vi "High_Voltage_Power_Supply_Control.vi"() -> ()   [LabVIEW 2016]
uses:
  High_Voltage_Power_Supply_Control_States.ctl
  <vilib>/Utility/file.llb/Write Delimited Spreadsheet (string).vi
panel:
  in  "File Path Control":path
  in  "STOP (T = stop)":bool
  in  "COM Port In":refnum<visa-resource-name>
  in  "Measuring speed (s)":dbl=1.0 caption="Time Target (s)"
  out "Emergency Stop (T = active)":bool
  out "Connection (T = active)":bool
  in  "Control Mode (T = CV, F = CC)":bool=TRUE
  out "CH2 CURRENT OUT (mA)":dbl format="%#_4f"
  out "CH2 VOLTAGE OUT (V)":i32
  out "CH1 CURRENT OUT (mA)":dbl format="%#_4f"
  out "CH1 VOLTAGE OUT (V)":i32
  in  "CH2 CURRENT SET (0...5 mA)":dbl=5.0 min=0.0 max=5.0 step=0.1 format="%_4f"
  in  "CH1 CURRENT SET (0...5 mA)":dbl=5.0 min=0.0 max=5.0 step=0.1 format="%_4f"
  in  "CH2 VOLTAGE SET (0...+2000 V)":i16 min=0 max=2000 step=100
  in  "CH1 VOLTAGE SET (-2000...0 V)":i16 min=-2000 max=0 step=100
  in  "CH2 ON/OFF (T = ON)":bool
  in  "CH1 ON/OFF (T = ON)":bool
  # "High Voltage Power Supply"
  # "CH1: -2000...0 V"
  # "CH2: 0...+2000 V"
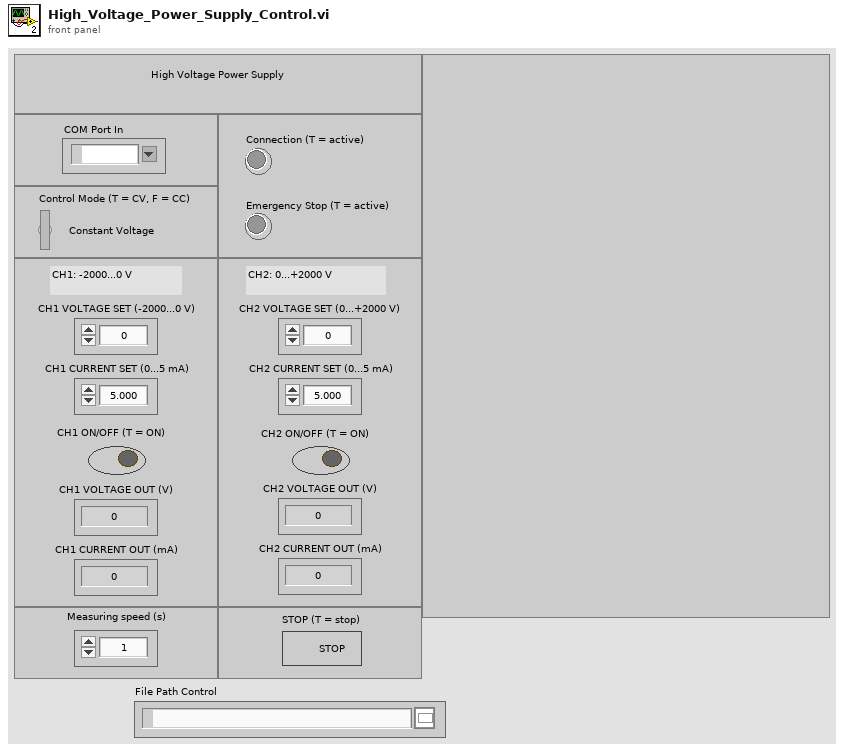
[diagram p1: front panel]
types:
  T1 = typedef "High_Voltage_Power_Supply_Control_States.ctl" = enum16{"CONTROL", "STOP", "INITIALISATION"}
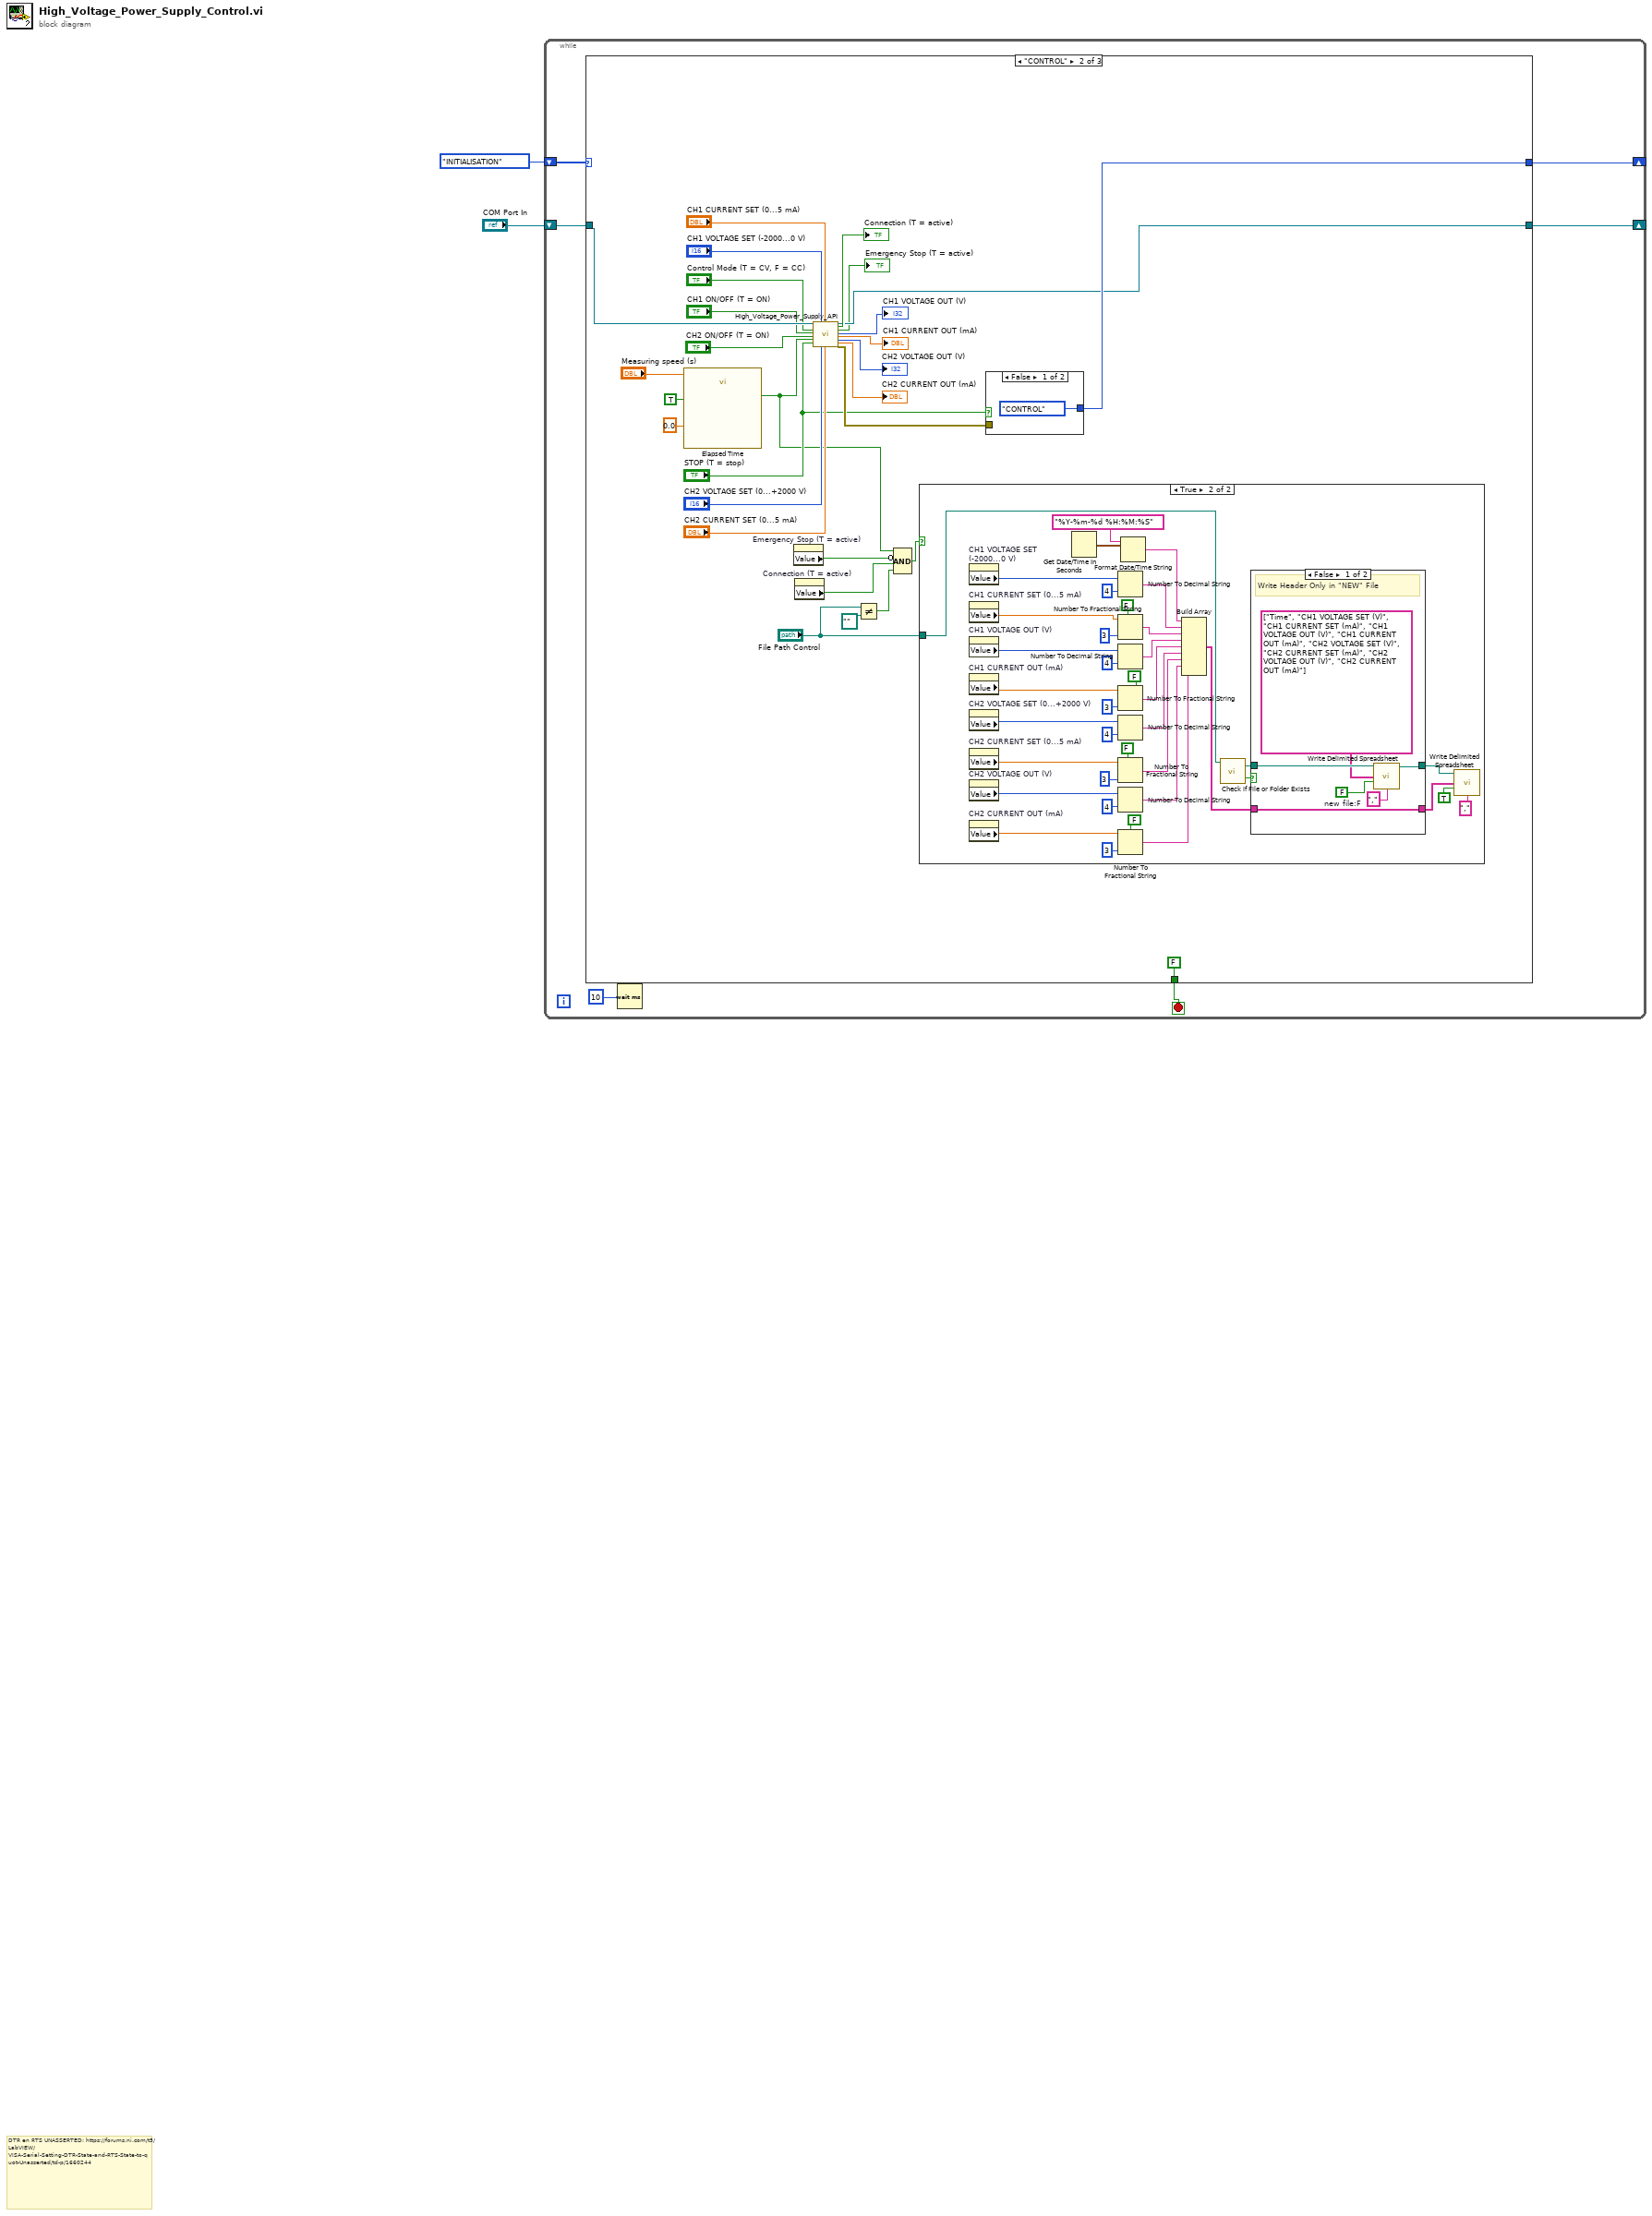
[diagram p0: block diagram]
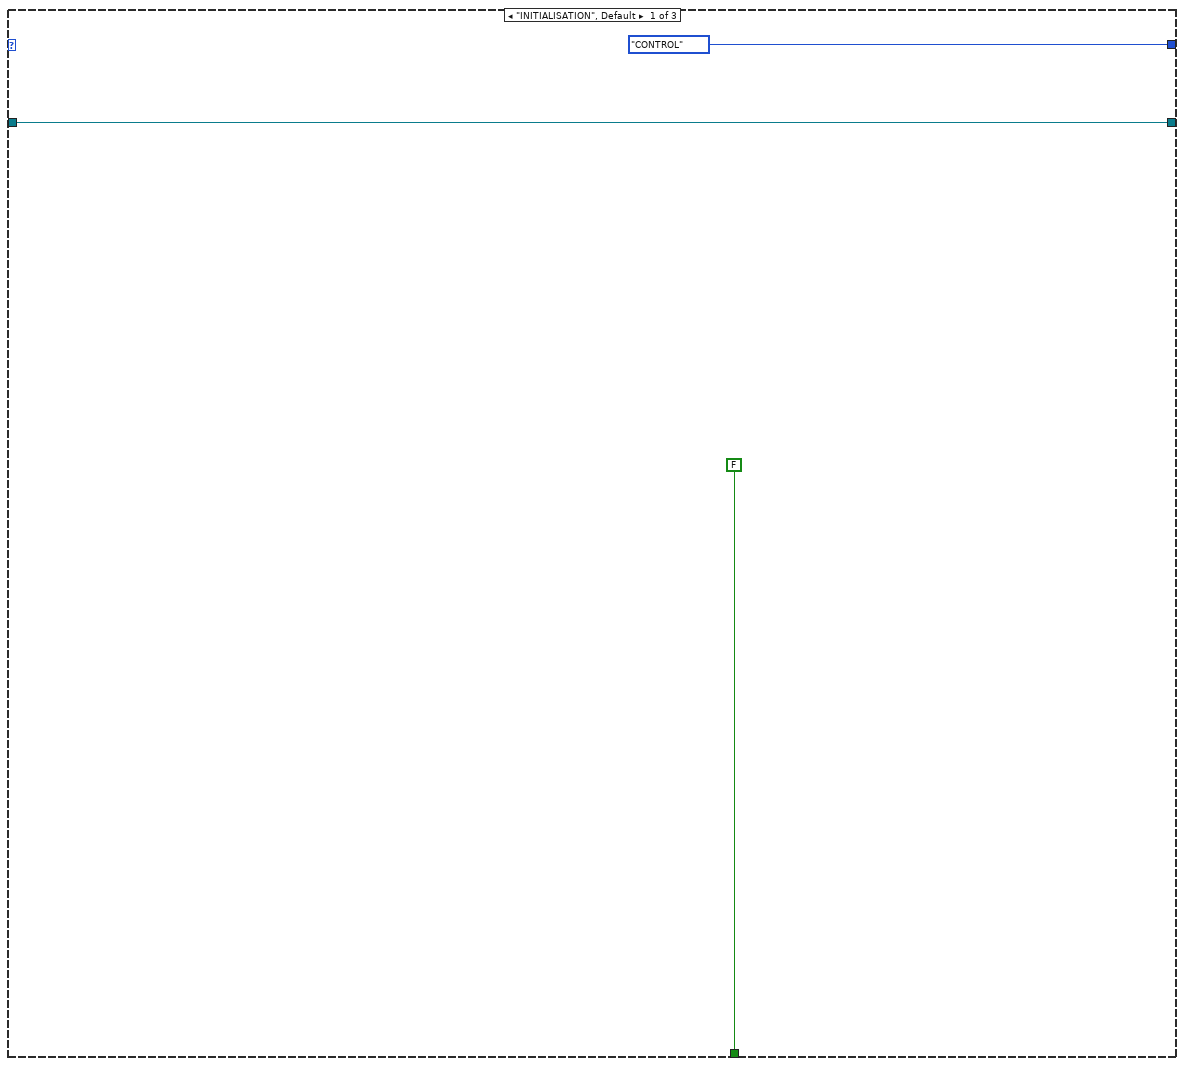
[diagram p2: hidden frame]
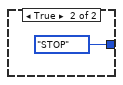
[diagram p5: hidden frame]
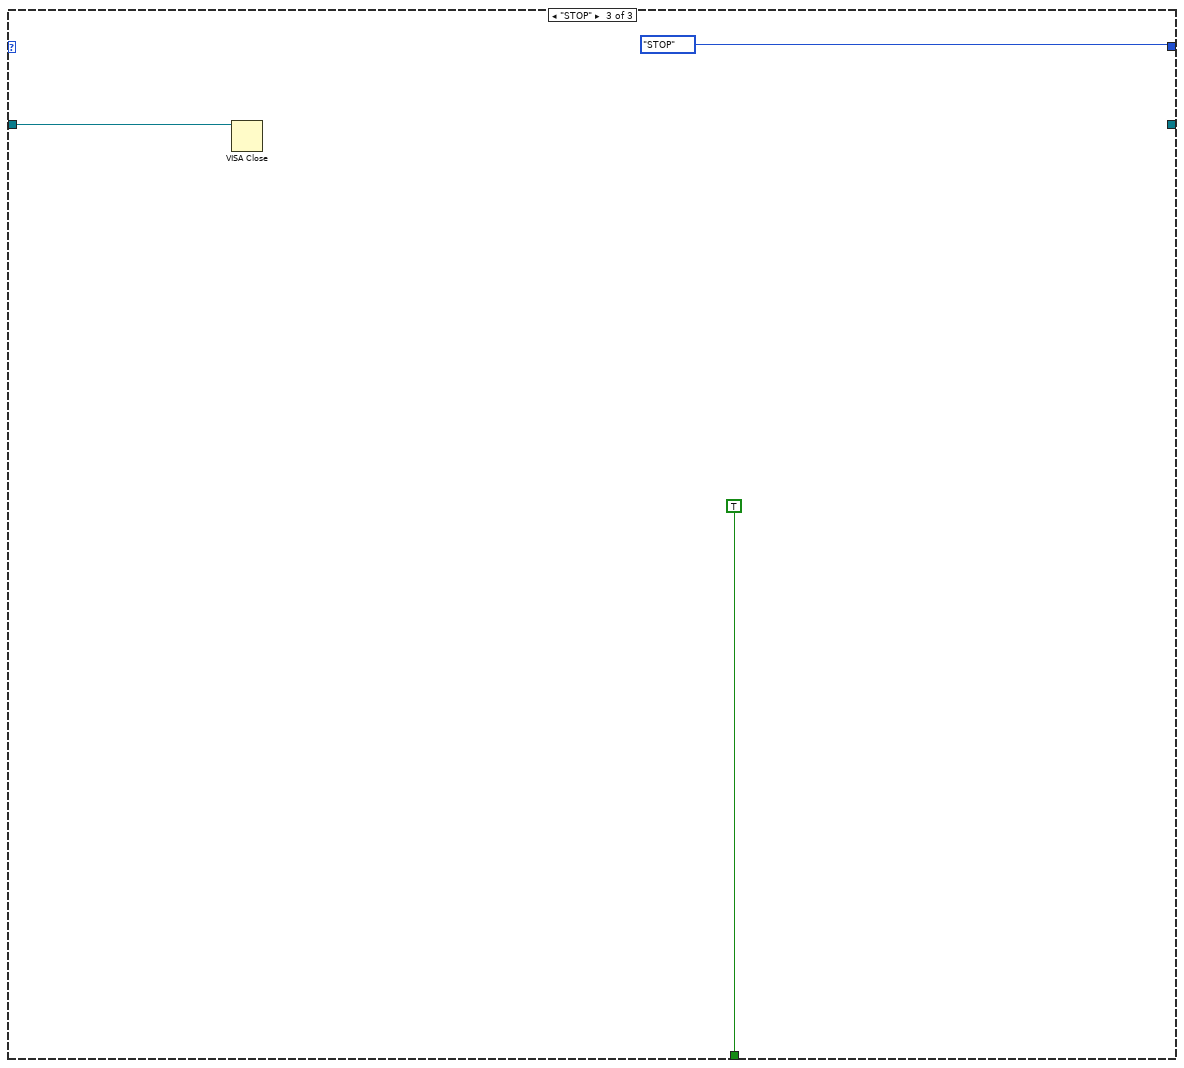
[diagram p6: hidden frame]
diagram:
  # "DTR en RTS UNASSERTED: https://forums.ni.com/t5/LabVIEW/VISA-Serial-Setting-DTR-State-and-RTS-State-to-quot-Unasserted/td-p/1660244"
  n1 = while {
    shift-right: [w6] -> _
    shift-left: High_Voltage_Power_Supply_Control_States."INITIALISATION" -> [w7]
    shift-right: [w4] -> _
    shift-left: "COM Port In" -> [w3]
    stop <- w5 stop-if-true
    n2 = case shown="\"CONTROL\"" w7 {
      tunnel: w3 -> [w9 w37 w92]
      tunnel: [High_Voltage_Power_Supply_Control_States."CONTROL" w39 High_Voltage_Power_Supply_Control_States."STOP"] -> w6
      tunnel: [FALSE FALSE TRUE] -> w5
      tunnel: [w9 w28 _] -> w4
      frame "INITIALISATION", Default {
      }
      frame "CONTROL" {
        n3 = call "Elapsed Time"("Time Target (s)"="Measuring speed (s)", "Auto Reset"=TRUE, "Set Start Time (s)"=0.0) -> ("Time has Elapsed"=w12:bool)  [unwired: 9 in, 7 out]
        n4 = property on="Emergency Stop (T = active)" class="Bool (strict)"() -> ("Value"=w16:bool)  [unwired: 2 in, 2 out]
        n5 = property on="Connection (T = active)" class="Bool (strict)"() -> ("Value"=w15:bool)  [unwired: 2 in, 2 out]
        n6 = call "High_Voltage_Power_Supply_API.vi"("COM Port In"=w37, "Control Mode (T = CV, F = CC)"="Control Mode (T = CV, F = CC)", "CH1 ON/OFF (T = ON)"="CH1 ON/OFF (T = ON)", "CH2 ON/OFF (T = ON)"="CH2 ON/OFF (T = ON)", "MEASURE (T = measure)"=w12, "STOP (T = stop)"="STOP (T = stop)", "CH1 VOLTAGE SET (-2000...0 V)"="CH1 VOLTAGE SET (-2000...0 V)", "CH2 VOLTAGE SET (0...+2000 V)"="CH2 VOLTAGE SET (0...+2000 V)", "CH1 CURRENT SET (0...5 mA)"="CH1 CURRENT SET (0...5 mA)", "CH2 CURRENT SET (0...5 mA)"="CH2 CURRENT SET (0...5 mA)") -> ("COM Port Out"=w28:refnum<visa-resource-name>, "Connection (T = active)"=→"Connection (T = active)":bool, "Emergency Stop (T = active)"=→"Emergency Stop (T = active)":bool, "CH1 VOLTAGE OUT (V)"=→"CH1 VOLTAGE OUT (V)":i32, "CH1 CURRENT OUT (mA)"=→"CH1 CURRENT OUT (mA)":dbl, "CH2 VOLTAGE OUT (V)"=→"CH2 VOLTAGE OUT (V)":i32, "CH2 CURRENT OUT (mA)"=→"CH2 CURRENT OUT (mA)":dbl, "error out"=w40:errorcluster)  [unwired: 10 in]
        n7 = Not Equal?(x="File Path Control", y=path "") -> (x != y?=w14:bool)
        n8 = Compound Arithmetic op=AND(w12, invert w16, w15, w14) -> (w13:bool)
        n9 = case shown="True" w13 {
          tunnel: "File Path Control" -> [_ w42]
          frame False {
          }
          frame True {
            n10 = property on="CH1 VOLTAGE SET (-2000...0 V)" class="DigNum (strict)"() -> ("Value"=w51:i16)  [unwired: 2 in, 2 out]
            n11 = property on="CH1 CURRENT SET (0...5 mA)" class="DigNum (strict)"() -> ("Value"=w50:dbl)  [unwired: 2 in, 2 out]
            n12 = property on="CH1 VOLTAGE OUT (V)" class="DigNum (strict)"() -> ("Value"=w49:i32)  [unwired: 2 in, 2 out]
            n13 = property on="CH1 CURRENT OUT (mA)" class="DigNum (strict)"() -> ("Value"=w48:dbl)  [unwired: 2 in, 2 out]
            n14 = property on="CH2 VOLTAGE SET (0...+2000 V)" class="DigNum (strict)"() -> ("Value"=w47:i16)  [unwired: 2 in, 2 out]
            n15 = property on="CH2 CURRENT SET (0...5 mA)" class="DigNum (strict)"() -> ("Value"=w46:dbl)  [unwired: 2 in, 2 out]
            n16 = property on="CH2 VOLTAGE OUT (V)" class="DigNum (strict)"() -> ("Value"=w45:i32)  [unwired: 2 in, 2 out]
            n17 = property on="CH2 CURRENT OUT (mA)" class="DigNum (strict)"() -> ("Value"=w44:dbl)  [unwired: 2 in, 2 out]
            n18 = Get Date/Time In Seconds() -> (seconds since 1Jan1904=w65:timestamp)
            n19 = Number To Decimal String(number=w51, width (-)=i16 4) -> (decimal integer string=w75:string)
            n20 = Number To Fractional String(use system decimal point (T)=FALSE, number=w50, precision (6)=i16 3) -> (F-format string=w76:string)  [unwired: 1 in]
            n21 = Number To Decimal String(number=w49, width (-)=i16 4) -> (decimal integer string=w74:string)
            n22 = Number To Fractional String(use system decimal point (T)=FALSE, number=w48, precision (6)=i16 3) -> (F-format string=w73:string)  [unwired: 1 in]
            n23 = Number To Decimal String(number=w47, width (-)=i16 4) -> (decimal integer string=w55:string)
            n24 = Number To Fractional String(use system decimal point (T)=FALSE, number=w46, precision (6)=i16 3) -> (F-format string=w54:string)  [unwired: 1 in]
            n25 = Number To Decimal String(number=w45, width (-)=i16 4) -> (decimal integer string=w53:string)
            n26 = Number To Fractional String(use system decimal point (T)=FALSE, number=w44, precision (6)=i16 3) -> (F-format string=w52:string)  [unwired: 1 in]
            n27 = Format Date/Time String(time format string (%c)="%Y-%m-%d %H:%M:%S", seconds (now)=w65) -> (date/time string=w64:string)  [unwired: 1 in]
            n28 = Build Array(w64, w75, w76, w74, w73, w55, w54, w53, w52) -> (w62:string[])
            n29 = call <vilib>:"Check if File or Folder Exists.vi"("path"=w42) -> ("file or folder exists?"=w43:bool, "dup path"=w79:path)  [unwired: 8 in, 1 out]
            n30 = case shown="False" w43 {
              tunnel: w79 -> [w85 w87]
              tunnel: [w84 w87] -> w78
              tunnel: w62 -> [w80 w86]
              tunnel: [w80 w86] -> w61
              frame False {
                w83 = FALSE  # new file:F
                # "Write Header Only in \"NEW\" File"
                n31 = call-poly <vilib>:"Write Delimited Spreadsheet.vi"("file path (dialog if empty)"=w85, "1D data"=string[] ["Time", "CH1 VOLTAGE SET (V)", "CH1 CURRENT SET (mA)", "CH1 VOLTAGE OUT (V)", "CH1 CURRENT OUT (mA)", "CH2 VOLTAGE SET (V)", "CH2 CURRENT SET (mA)", "CH2 VOLTAGE OUT (V)", "CH2 CURRENT OUT (mA)"], "append to file? (new file:F)"=w83, "delimiter (\\t)"="," ("delimiter (\\t)")) -> ("new file path (Not A Path if cancelled)"=w84:path)  [unwired: 10 in, 1 out]
              }
              frame True {
                # "File alreade exists. Don't need to write header"
              }
            }
            n32 = call-poly <vilib>:"Write Delimited Spreadsheet.vi"("file path (dialog if empty)"=w78, "1D data"=w61, "append to file? (new file:F)"=TRUE ("append to file:T"), "delimiter (\\t)"="," ("delimiter (\\t)")) -> ()  [unwired: 10 in, 2 out]
          }
        }
        n33 = case shown="False" "STOP (T = stop)" {
          tunnel: w40 -> [_ _]
          tunnel: [High_Voltage_Power_Supply_Control_States."CONTROL" High_Voltage_Power_Supply_Control_States."STOP"] -> w39
          frame False {
          }
          frame True {
          }
        }
      }
      frame "STOP" {
        n34 = VISA Close(VISA resource name=w92) -> ()  [unwired: 1 in, 1 out]
      }
    }
    n35 = Wait (ms)(milliseconds to wait=u32 10) -> ()  [unwired: 1 out]
  }
